vi "count Cyclone Images.vi"(8 "error in":errorcluster, 11 "cycloneHandle":u32) -> (0 "error out":errorcluster, 3 "function return":u32)   [LabVIEW 2021, in "CycloneControlSDK.lvlib"]
doc: "extern \"C\" uint32_t _cdecl countCycloneImages(uint32_t cycloneHandle);"
uses:
  CycloneControlSDK.lvlib
  CycloneControlSDK_64.dll
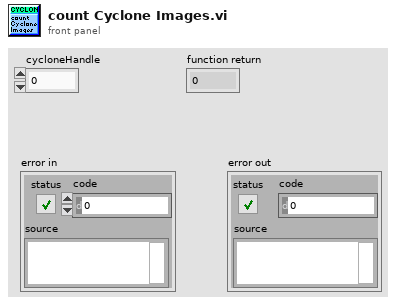
[diagram p1: front panel]
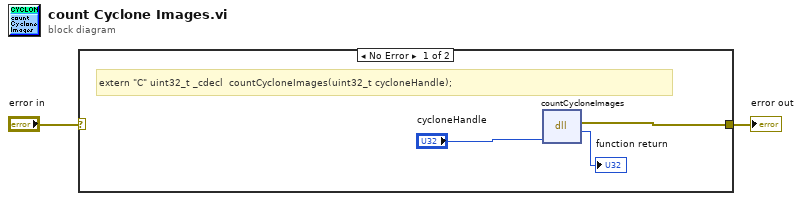
[diagram p0: block diagram]
diagram:
  n1 = case shown="No Error" "error in" {
    selector: "error in" -> [_ w6]
    tunnel: [w3 w6] -> w1
    frame No Error {
      # "extern \"C\" uint32_t _cdecl  countCycloneImages(uint32_t cycloneHandle);"
      n2 = dll-call lib="C:/PEMicro/cyclone/cycloneControl/controlsdk/examples/labview2018/user.lib/CycloneControlSDK/CycloneControlSDK_64.dll" fn="countCycloneImages"("cycloneHandle"="cycloneHandle") -> (error out=w3:errorcluster, "return type"=→"function return":u32)  [unwired: 4 in, 1 out]
    }
    frame Error {
    }
  }
  "error out" <- w1
